vi "GetHistogramFromXYgraph.vi"(6 "Numeric":i32, 9 "image  IN":dbl[][](graph), 11 "Statistics (n-1)":T1) -> (3 "Statistics (n)":cluster{dbl[][], dbl[][]})   [LabVIEW 2018]
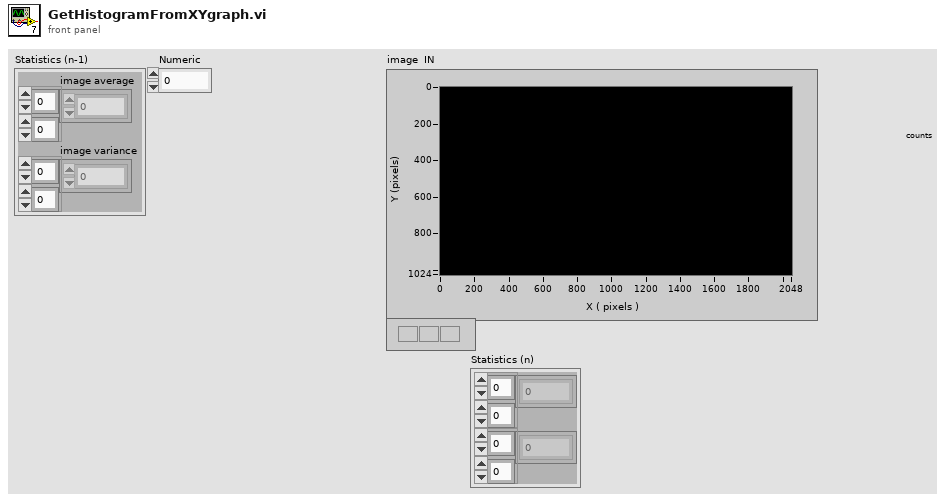
[diagram p1: front panel]
types:
  T1 = cluster{"image average":dbl[][], "image variance":dbl[][]}
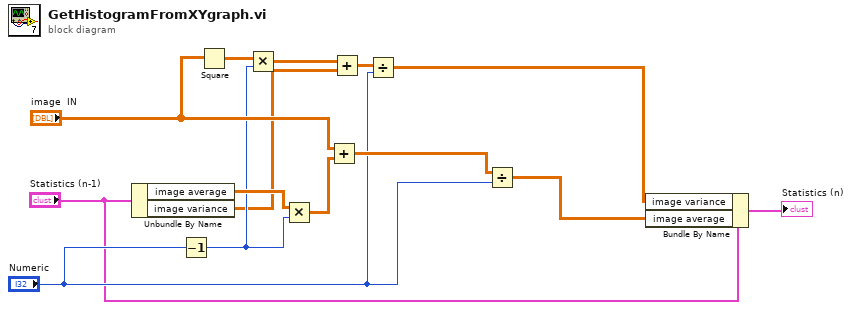
[diagram p0: block diagram]
diagram:
  n1 = Unbundle By Name("Statistics (n-1)") -> ("image average"=w14:dbl[][], "image variance"=w7:dbl[][])
  n2 = Decrement(x="Numeric") -> (x-1=w9:i32)
  n3 = Square(x="image  IN") -> (x^2=w10:dbl[][])
  n4 = Multiply(x=w10, y=w9) -> (x*y=w8:dbl[][])
  n5 = Multiply(x=w14, y=w9) -> (x*y=w13:dbl[][])
  n6 = Add(x="image  IN", y=w13) -> (x+y=w12:dbl[][])
  n7 = Add(x=w8, y=w7) -> (x+y=w6:dbl[][])
  n8 = Divide(x=w6, y="Numeric") -> (x/y=w2:dbl[][])
  n9 = Divide(x=w12, y="Numeric") -> (x/y=w1:dbl[][])
  n10 = Bundle By Name(cluster="Statistics (n-1)", "image variance"=w2, "image average"=w1) -> (→"Statistics (n)":T1)
